vi "TDMS_STR_Array to file.vi"(5 "Interval":T1=enum."Daily", 6 "channel name(s) in":string[](array[string])=["Time", "Distance"], 7 "group name in (Untitled)":string="SonarAlt", 8 "error in (no error)":errorcluster, 9 "Data":string[](array[string]), 10 "FilePrefix":string, 11 "Base path":path) -> (0 "error out":errorcluster, 3 "sonic file out":refnum<k34>)   [LabVIEW 2025]
uses:
  Enum_FileNewInterval.ctl
  4eaa4cfa-5103-44e1-8cfa-05a335443445.vi
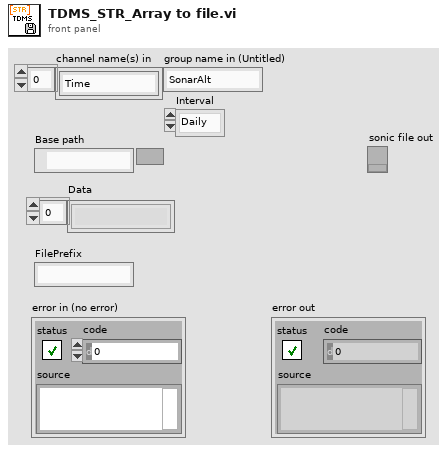
[diagram p1: front panel]
types:
  T1 = typedef "Enum_FileNewInterval.ctl" = enum16{"2 Min", "10 Min", "Hourly", "Daily", "Weekly", "Monthly"}
  T2 = enum16{"open", "open or create", "create or replace", "create", "open (read-only)"}
  T3 = typedef "LVDateTimeRec.ctl" = cluster{"fractional second":dbl, "second":i32, "minute":i32, "hour":i32, "day of month":i32, "month":i32, "year":i32, "day of week":i32, "day of year":i32, "DST":i32}
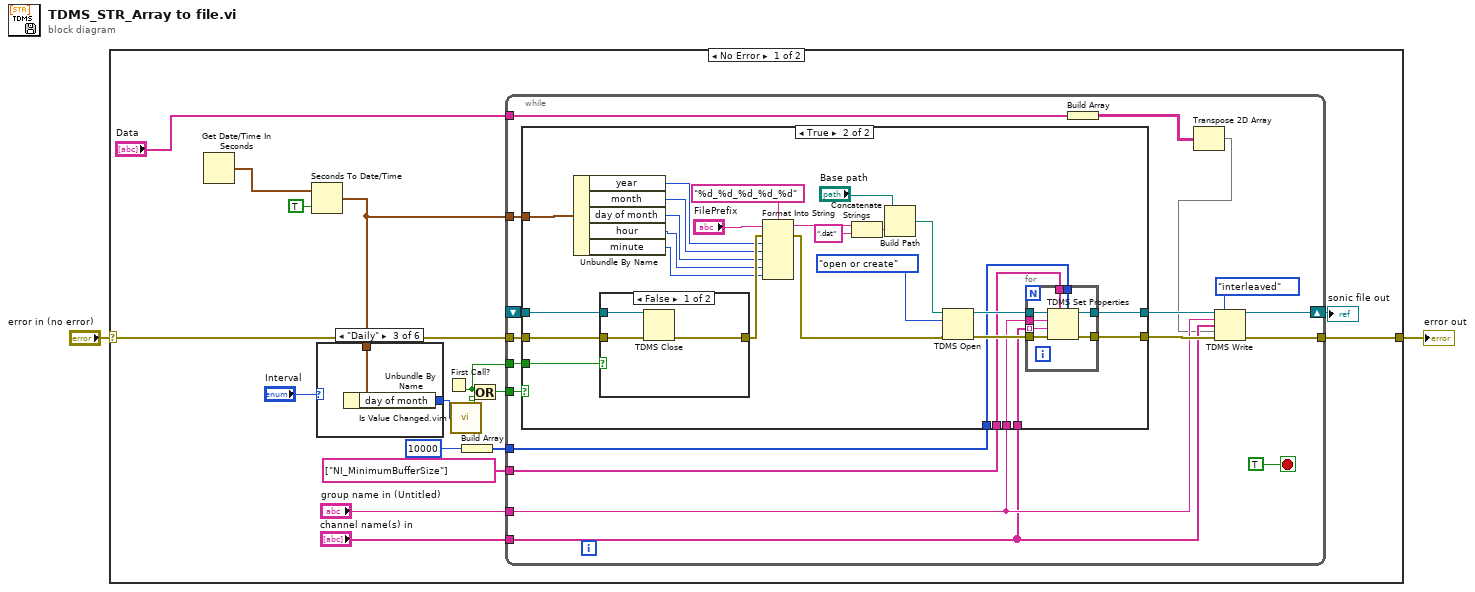
[diagram p0: block diagram]
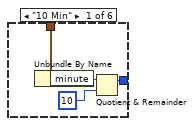
[diagram p2: hidden frame]
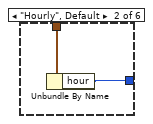
[diagram p3: hidden frame]
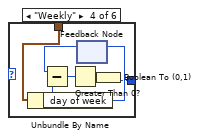
[diagram p4: hidden frame]
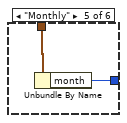
[diagram p5: hidden frame]
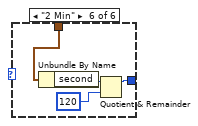
[diagram p6: hidden frame]
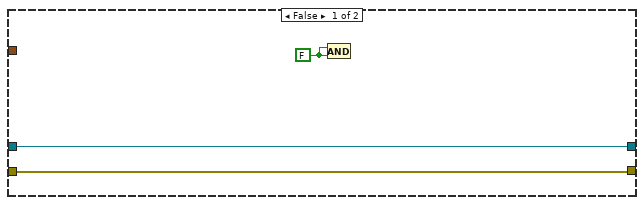
[diagram p7: hidden frame]
diagram:
  n1 = case shown="No Error" "error in (no error)" {
    selector: "error in (no error)" -> [w15 w100]
    tunnel: [w17 w100] -> w2
    frame No Error {
      n2 = Get Date/Time In Seconds() -> (seconds since 1Jan1904=w6:timestamp)
      n3 = Seconds To Date/Time(time stamp (now)=w6, to UTC (F)=TRUE) -> (date time rec=w5:T3)
      n4 = case shown="\"Daily\"" "Interval" {
        tunnel: w5 -> [w23 w25 w27 w33 w35 w37]
        tunnel: [w20 w24 w26 w28 w34 w36] -> w4
        frame "10 Min" {
          n5 = Unbundle By Name(w23) -> ("minute"=w22:i32)
          n6 = Quotient & Remainder(x=w22, y=10) -> (floor(x/y)=w20:i32)  [unwired: 1 out]
        }
        frame "Hourly", Default {
          n7 = Unbundle By Name(w25) -> ("hour"=w24:i32)
        }
        frame "Daily" {
          n8 = Unbundle By Name(w27) -> ("day of month"=w26:i32)
        }
        frame "Weekly" {
          n9 = Unbundle By Name(w33) -> ("day of week"=w31:i32)
          n10 = feedback-in #1(w31) -> ()
          n11 = feedback #1() -> (w32:i32)  [unwired: 1 in]
          n12 = Subtract(x=w32, y=w31) -> (x-y=w30:i32)
          n13 = Greater Than 0?(x=w30) -> (x > 0?=w29:bool)
          n14 = Boolean To (0,1)(Boolean=w29) -> (0, 1=w28:i16)
        }
        frame "Monthly" {
          n15 = Unbundle By Name(w35) -> ("month"=w34:i32)
        }
        frame "2 Min" {
          n16 = Unbundle By Name(w37) -> ("second"=w39:i32)
          n17 = Quotient & Remainder(x=w39, y=120) -> (x-y*floor(x/y)=w36:i32)  [unwired: 1 out]
        }
      }
      n18 = First Call?() -> (First Call?: T/F=w18:bool)
      n19 = call "Is Value Changed.vim"("value"=w4) -> ("changed or first call?"=w3:bool)
      n20 = Build Array(10000) -> (w9:i32[])
      n21 = Or(x=w18, y=w3) -> (x .or. y?=w19:bool)
      n22 = while {
        tunnel: w19 -> [w57]
        shift-right: [w49] -> w16
        shift-left: _ -> [w56]
        tunnel: w18 -> [w55]
        tunnel: "Data" -> [w42]
        tunnel: [w48] -> w17
        tunnel: w15 -> [w54]
        tunnel: w5 -> [w52]
        tunnel: "channel name(s) in" -> [w43]
        tunnel: "group name in (Untitled)" -> [w44]
        tunnel: w9 -> [w46]
        tunnel: string[] ["NI_MinimumBufferSize"] ("Channel Names") -> [w45]
        stop <- TRUE stop-if-true
        n23 = case shown="True" w57 {
          tunnel: [w60 w66] -> w51
          tunnel: w56 -> [w60 w79]
          tunnel: w55 -> [_ w80]
          tunnel: [w59 w65] -> w50
          tunnel: w54 -> [w59 w78]
          tunnel: w52 -> [_ w69]
          tunnel: w46 -> [_ w64]
          tunnel: w45 -> [_ w63]
          tunnel: w44 -> [_ w62]
          tunnel: w43 -> [_ w61]
          frame False {
            w58 = FALSE ("y")
            n24 = And(x=w58, y=w58) -> ()  [unwired: 1 out]
          }
          frame True {
            n25 = Unbundle By Name(w69) -> ("year"=w77:i32, "month"=w76:i32, "day of month"=w75:i32, "hour"=w72:i32, "minute"=w71:i32)
            n26 = case shown="False" w80 {
              tunnel: w79 -> [w98 _]
              tunnel: [w97 w99] -> w87
              tunnel: w78 -> [w96 w99]
              frame False {
                n27 = TDMS Close(8:w96, 11:w98) -> (0:w97:errorcluster)  [unwired: 1 out]
              }
              frame True {
              }
            }
            n28 = Format Into String(format string="%d_%d_%d_%d_%d", initial string="FilePrefix", error in=w87, w77, w76, w75, w72, w71) -> (resulting string=w86:string, error out=w70:errorcluster)
            n29 = Concatenate Strings(w86, ".dat" ("string")) -> (w83:string)
            n30 = Build Path(base path="Base path", name or relative path=w83) -> (appended path=w82:path)
            n31 = TDMS Open(8:w70, 10:T2."open or create" ("operation (0:open)"), 11:w82) -> (0:w68:errorcluster, 3:w67:refnum<k34>)  [unwired: 4 in]
            n32 = for {
              tunnel: w67 -> [w95]
              tunnel: [w94] -> w66
              tunnel: w68 -> [w93]
              tunnel: [w92] -> w65
              tunnel: w63 -> [w91]
              tunnel: w64 -> [w90]
              tunnel: w62 -> [w89]
              tunnel: w61 -> [w88] mode=indexing
              n33 = TDMS Set Properties(5:w90, 7:w91, 8:w93, 9:w88, 10:w89, 11:w95) -> (0:w92:errorcluster, 3:w94:refnum<k34>)  [unwired: 2 out]
            }
          }
        }
        n34 = Build Array(w42) -> (w41:string[][])
        n35 = Transpose 2D Array(2D array=w41) -> (transposed array=w40:string[][])
        n36 = TDMS Write(0:w51, 1:enum16{"decimated", "interleaved"}."interleaved" ("data layout (0:decimated)"), 5:w44, 7:w43, 9:w40, 11:w50) -> (4:w49:refnum<k34>, 15:w48:errorcluster)  [unwired: 2 out]
      }
      "sonic file out" <- w16
    }
    frame Error {
    }
  }
  "error out" <- w2
